vi "Async VI Control_Create Trigger.vi"(6 "This VI":refnum<vi>, 8 "error in (no error)":errorcluster) -> (0 "error out":errorcluster)   [LabVIEW 2021, in "CANOpen Addon Engine.lvlib"]
uses:
  CANOpen Addon Engine.lvlib
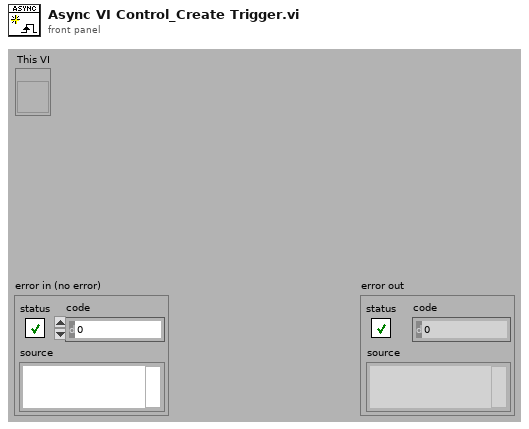
[diagram p1: front panel]
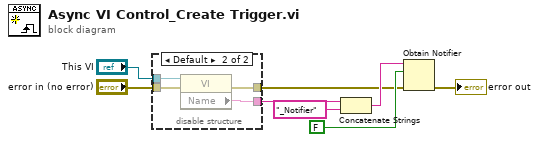
[diagram p0: block diagram]
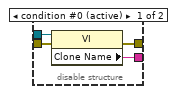
[diagram p2: hidden frame]
diagram:
  n1 = disable-structure shown="Default" {
    disable-tunnel: "error in (no error)" -> [w12 w16]
    disable-tunnel: "This VI" -> [w11 w15]
    disable-tunnel: [w10 w14] -> w5
    disable-tunnel: [w9 w13] -> w1
    frame condition #0 (active) {
      n2 = property class="VI"(reference=w11, error in=w12) -> (error out=w9:errorcluster, "Clone Name"=w10:string)  [unwired: 1 out]
    }
    frame condition #1 {
      n3 = property class="VI"(reference=w15, error in=w16) -> (error out=w13:errorcluster, "Name"=w14:string)  [unwired: 1 out]
    }
  }
  n4 = Concatenate Strings(w5, "_Notifier" ("name (unnamed)")) -> (w3:string)
  n5 = Obtain Notifier(name (unnamed)=w3, notification data type=FALSE, error in (no error)=w1) -> (error out=→"error out":errorcluster)  [unwired: 1 in, 2 out]
